vi "Single channel reverb ver2.vi"(8 "tail length":i32, 9 "fade gain":dbl, 10 "fade delay":i32, 11 "data in":waveform(dbl)) -> (3 "data out":waveform(dbl))   [LabVIEW 2023]
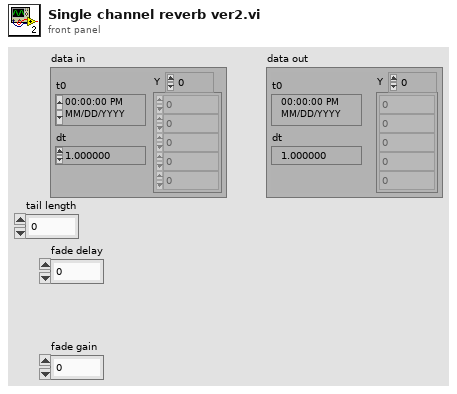
[diagram p1: front panel]
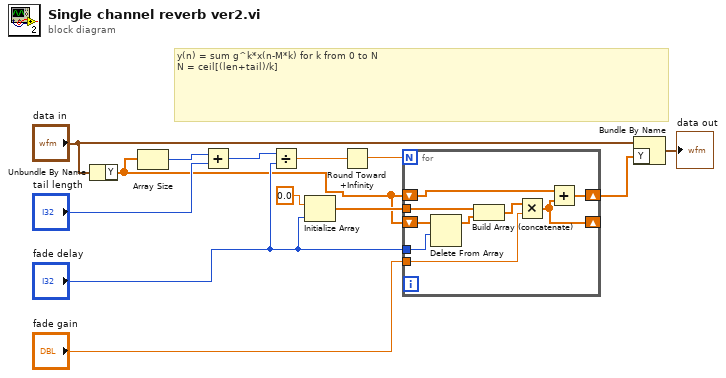
[diagram p0: block diagram]
diagram:
  # "y(n) = sum g^k*x(n-M*k) for k from 0 to N\nN = ceil[(len+tail)/k]"
  n1 = Unbundle By Name("data in") -> ("Y"=w1:dbl[])
  n2 = Array Size(array=w1) -> (size(s)=w10:i32)
  n3 = Add(x=w10, y="tail length") -> (x+y=w9:i32)
  n4 = Divide(x=w9, y="fade delay") -> (x/y=w8:dbl)
  n5 = Initialize Array(0.0 ("element"), "fade delay") -> (w4:dbl[])
  n6 = Round Toward +Infinity(x=w8) -> (ceil(x): smallest int >= x=w7:dbl)
  n7 = for {
    N: w7 -> [_]
    shift-right: [w21] -> w2
    shift-left: w1 -> [w22]
    tunnel: "fade delay" -> [w16]
    tunnel: w4 -> [w19]
    shift-right: [w14] -> _
    shift-left: w1 -> [w17]
    tunnel: "fade gain" -> [w15]
    n8 = Delete From Array(array=w17, length=w16) -> (array with subset deleted=w20:dbl[])  [unwired: 1 in, 1 out]
    n9 = Build Array (concatenate)(w19, w20) -> (w18:dbl[])
    n10 = Multiply(x=w18, y=w15) -> (x*y=w14:dbl[])
    n11 = Add(x=w22, y=w14) -> (x+y=w21:dbl[])
  }
  n12 = Bundle By Name(cluster="data in", "Y"=w2) -> (→"data out":waveform(dbl))
